vi "Parse SNMP Tuple.vi"(8 "error in (no error)":errorcluster, 11 "SNMP Packet In":u8[](array[numeric]) format="%.0x") -> (0 "error out":errorcluster, 1 "Data Out":T1, 2 "Data Type":u8, 3 "SNMP Packet Out":u8[](array[numeric]) format="%.0x", 4 "Data As String":string)   [LabVIEW 2017]
doc: "This VI is used to parse a single data tuple into its appropriate data type. The data value is returned in a cluster which contains the three basic data types which comprise SNMP data. These are a numberic value (UINT32), an ASCII string and a byte array. The data is returned in the appropriate element of the cluster based on the SNMP data type of the item. The data value is also returned as an ASCII string."
panel:
  out "Output Array":u8[](array[numeric]) format="%.0x"
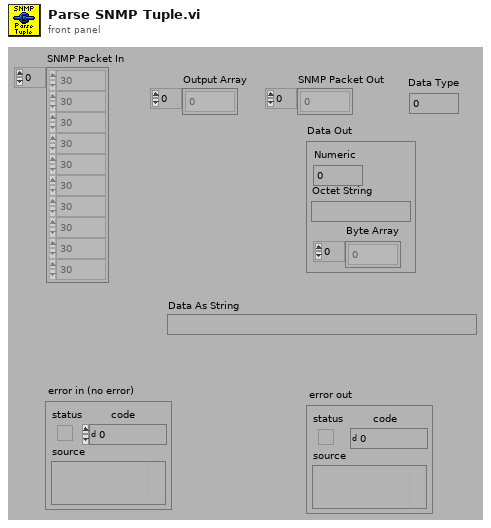
[diagram p1: front panel]
types:
  T1 = cluster{"Numeric":u32, "Octet String":string, "Byte Array":u8[]}
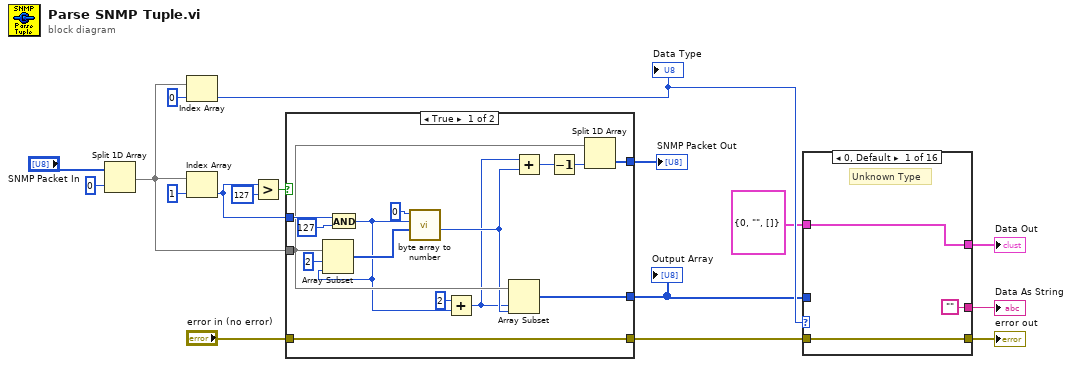
[diagram p0: block diagram]
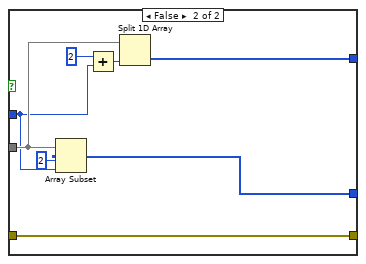
[diagram p2: hidden frame]
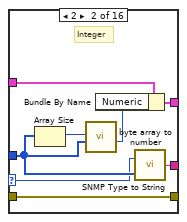
[diagram p3: hidden frame]
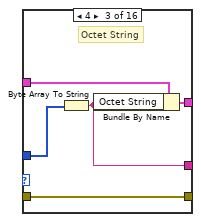
[diagram p4: hidden frame]
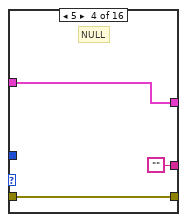
[diagram p5: hidden frame]
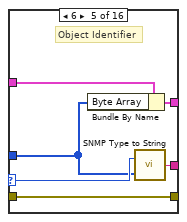
[diagram p6: hidden frame]
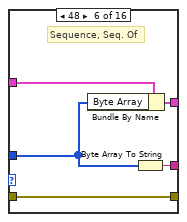
[diagram p7: hidden frame]
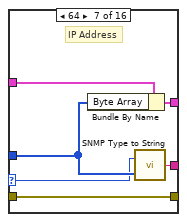
[diagram p8: hidden frame]
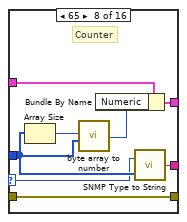
[diagram p9: hidden frame]
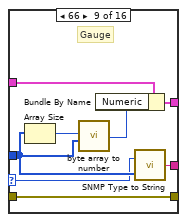
[diagram p10: hidden frame]
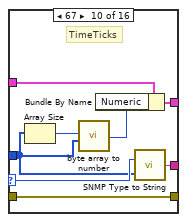
[diagram p11: hidden frame]
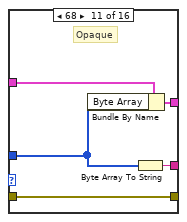
[diagram p12: hidden frame]
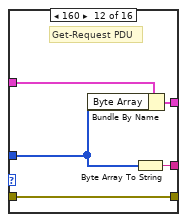
[diagram p13: hidden frame]
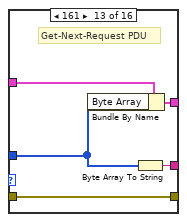
[diagram p14: hidden frame]
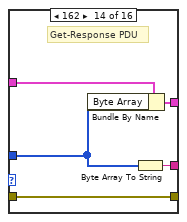
[diagram p15: hidden frame]
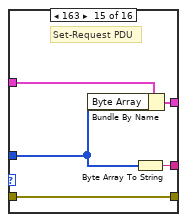
[diagram p16: hidden frame]
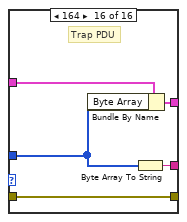
[diagram p17: hidden frame]
diagram:
  n1 = Split 1D Array(array="SNMP Packet In", index=0) -> (second subarray=w8:u8[])  [unwired: 1 out]
  n2 = Index Array(array=w8, index=0 ("Index")) -> (element=w17:u8)
  "Data Type" <- w17
  n3 = Index Array(array=w8, index=1 ("Index")) -> (element=w12:u8)
  n4 = Greater?(x=w12, y=u8 127) -> (0:w13:bool)
  n5 = case shown="True" w13 {
    tunnel: w12 -> [w32 w37]
    tunnel: w8 -> [w29 w38]
    tunnel: [w26 w34] -> w2
    tunnel: [w25 w35] -> w11
    tunnel: [w20 w33] -> w4
    tunnel: "error in (no error)" -> [w20 w33]
    frame True {
      n6 = And(x=w32, y=u8 127) -> (x .and. y?=w22:u8)
      n7 = Array Subset(array=w29, index=2 ("Array Index"), length=w22) -> (w23:u8[])
      n8 = call "byte array to number.vi"("Byte Array"=w23, "Byte Length"=w22, "Start Value"=u32 0) -> ("Number"=w19:u32)  [unwired: 1 in, 7 out]
      n9 = Add(x=u8 2, y=w22) -> (x+y=w18:u8)
      n10 = Array Subset(array=w29, index=w18, length=w19) -> (w26:u8[])
      n11 = Add(x=w18, y=w19) -> (x+y=w27:u32)
      n12 = Decrement(x=w27) -> (x-1=w24:u32)
      n13 = Split 1D Array(array=w29, index=w24) -> (second subarray=w25:u8[])  [unwired: 1 out]
    }
    frame False {
      n14 = Array Subset(array=w38, index=2 ("Array Index"), length=w37) -> (w34:u8[])
      n15 = Add(x=u8 2, y=w37) -> (x+y=w39:u8)
      n16 = Split 1D Array(array=w38, index=w39) -> (second subarray=w35:u8[])  [unwired: 1 out]
    }
  }
  "Output Array" <- w2
  "SNMP Packet Out" <- w11
  n17 = case shown="0, Default" w17 {
    selector: w17 -> [_ w44 _ _ w61 _ w71 w78 w86 w95 _ _ _ _ _ _]
    tunnel: w2 -> [_ w45 w56 _ w60 w66 w73 w79 w87 w94 w101 w106 w112 w117 w121 w127]
    tunnel: T1 {"Numeric"=0, "Octet String"="", "Byte Array"=[]} ("Data Out") -> [w43 w51 w55 w59 w64 w70 w76 w84 w92 w100 w105 w110 w115 w120 w125 w130]
    tunnel: [w43 w49 w54 w59 w65 w69 w75 w82 w90 w99 w104 w109 w114 w119 w124 w129] -> w9
    tunnel: [w42 w47 w53 w58 w63 w68 w74 w80 w88 w97 w103 w108 w113 w118 w123 w128] -> w3
    tunnel: w4 -> [w42 w47 w53 w58 w63 w68 w74 w80 w88 w97 w103 w108 w113 w118 w123 w128]
    tunnel: ["" w46 w52 "" w62 w67 w72 w77 w85 w93 w102 w107 w111 w116 w122 w126] -> w1
    frame 0, Default {
      # "Unknown Type"
    }
    frame 2 {
      # "Integer"
      n18 = Array Size(array=w45) -> (size(s)=w48:i32)
      n19 = call "byte array to number.vi"("Byte Array"=w45, "Byte Length"=w48) -> ("Number"=w50:u32)  [unwired: 2 in, 7 out]
      n20 = Bundle By Name(cluster=w51, "Numeric"=w50) -> (w49:T1)
      n21 = call "SNMP Type to String.vi"("Data"=w45, "Type"=w44) -> ("TypeAsString"=w46:string)
    }
    frame 4 {
      # "Octet String"
      n22 = Byte Array To String(unsigned byte array=w56) -> (string=w52:string)
      n23 = Bundle By Name(cluster=w55, "Octet String"=w52) -> (w54:T1)
    }
    frame 5 {
      # "NULL"
    }
    frame 6 {
      # "Object Identifier"
      n24 = Bundle By Name(cluster=w64, "Byte Array"=w60) -> (w65:T1)
      n25 = call "SNMP Type to String.vi"("Data"=w60, "Type"=w61) -> ("TypeAsString"=w62:string)
    }
    frame 48 {
      # "Sequence, Seq. Of"
      n26 = Bundle By Name(cluster=w70, "Byte Array"=w66) -> (w69:T1)
      n27 = Byte Array To String(unsigned byte array=w66) -> (string=w67:string)
    }
    frame 64 {
      # "IP Address"
      n28 = Bundle By Name(cluster=w76, "Byte Array"=w73) -> (w75:T1)
      n29 = call "SNMP Type to String.vi"("Data"=w73, "Type"=w71) -> ("TypeAsString"=w72:string)
    }
    frame 65 {
      # "Counter"
      n30 = Array Size(array=w79) -> (size(s)=w81:i32)
      n31 = call "byte array to number.vi"("Byte Array"=w79, "Byte Length"=w81) -> ("Number"=w83:u32)  [unwired: 2 in, 7 out]
      n32 = Bundle By Name(cluster=w84, "Numeric"=w83) -> (w82:T1)
      n33 = call "SNMP Type to String.vi"("Data"=w79, "Type"=w78) -> ("TypeAsString"=w77:string)
      n34 = call "byte array to number.vi"() -> ()  [unwired: 3 in, 9 out]
    }
    frame 66 {
      # "Gauge"
      n35 = Array Size(array=w87) -> (size(s)=w89:i32)
      n36 = call "byte array to number.vi"("Byte Array"=w87, "Byte Length"=w89) -> ("Number"=w91:u32)  [unwired: 2 in, 7 out]
      n37 = Bundle By Name(cluster=w92, "Numeric"=w91) -> (w90:T1)
      n38 = call "SNMP Type to String.vi"("Data"=w87, "Type"=w86) -> ("TypeAsString"=w85:string)
      n39 = call "byte array to number.vi"() -> ()  [unwired: 3 in, 9 out]
    }
    frame 67 {
      # "TimeTicks"
      n40 = Array Size(array=w94) -> (size(s)=w98:i32)
      n41 = call "byte array to number.vi"("Byte Array"=w94, "Byte Length"=w98) -> ("Number"=w96:u32)  [unwired: 2 in, 7 out]
      n42 = Bundle By Name(cluster=w100, "Numeric"=w96) -> (w99:T1)
      n43 = call "SNMP Type to String.vi"("Data"=w94, "Type"=w95) -> ("TypeAsString"=w93:string)
    }
    frame 68 {
      # "Opaque"
      n44 = Bundle By Name(cluster=w105, "Byte Array"=w101) -> (w104:T1)
      n45 = Byte Array To String(unsigned byte array=w101) -> (string=w102:string)
    }
    frame 160 {
      # "Get-Request PDU"
      n46 = Bundle By Name(cluster=w110, "Byte Array"=w106) -> (w109:T1)
      n47 = Byte Array To String(unsigned byte array=w106) -> (string=w107:string)
    }
    frame 161 {
      # "Get-Next-Request PDU"
      n48 = Bundle By Name(cluster=w115, "Byte Array"=w112) -> (w114:T1)
      n49 = Byte Array To String(unsigned byte array=w112) -> (string=w111:string)
    }
    frame 162 {
      # "Get-Response PDU"
      n50 = Bundle By Name(cluster=w120, "Byte Array"=w117) -> (w119:T1)
      n51 = Byte Array To String(unsigned byte array=w117) -> (string=w116:string)
    }
    frame 163 {
      # "Set-Request PDU"
      n52 = Bundle By Name(cluster=w125, "Byte Array"=w121) -> (w124:T1)
      n53 = Byte Array To String(unsigned byte array=w121) -> (string=w122:string)
    }
    frame 164 {
      # "Trap PDU"
      n54 = Bundle By Name(cluster=w130, "Byte Array"=w127) -> (w129:T1)
      n55 = Byte Array To String(unsigned byte array=w127) -> (string=w126:string)
    }
  }
  "error out" <- w3
  "Data Out" <- w9
  "Data As String" <- w1
